vi "Single Tone Multi Ch Audio Measurements.vi"(8 "error in":errorcluster, 9 "units":T1, 10 "measurement settings":T3={"Band start"=20.0, "Band stop"=20000.0, "Amplitude"=1.0, "Frequency"=1000.0, "Full scale range"=3.16}, 11 "waveforms":waveform(dbl)[](array[waveform])) -> (0 "error out":errorcluster, 1 "spectra":cluster{"x0":dbl, "dx":dbl, "magnitude":dbl[]}[](array[cluster]), 2 "waveforms":waveform(dbl)[](array[waveform]), 3 "results":T2(array[cluster]))   [LabVIEW 2021]
uses:
  controls/Single Tone Measurement Settings.ctl
  controls/Single Tone Units.ctl
  <vilib>/addons/_NISVFA/_Shared subVIs/Common/SVL Set dB Reference (N Ch - 1 Ref).vi
  <vilib>/addons/Sound and Vibration/svt_Single Tone Measurements/SVT Spurious Free Dynamic Range (Frequency) (1 Ch).vi
  <vilib>/addons/_NISVFA/_Spectrum Processing/SVFA Unit Conversion (Complex) (1 Ch).vi
  <vilib>/addons/_NISVFA/_Spectrum Processing/SVFA Get Spectrum Subset (1 Ch).vi
  <vilib>/addons/_NISVFA/_Shared subVIs/Common/SVL Set dB Reference (1 Ch).vi
  <vilib>/addons/_NISVFA/_Spectrum Processing/SVFA Get Spectrum Subset (Complex) (1 Ch).vi
  <vilib>/addons/_NISVFA/_Shared subVIs/Common/svc_Window Parameters.vi
  <vilib>/addons/_NISVFA/_Shared subVIs/Common/svc_Extract Single Tone Information (complex).vi
  <vilib>/addons/_NISVFA/_Shared subVIs/Common/svc_Check Frequency Range in Spectrum.vi
  <vilib>/addons/_NISVFA/_Spectrum Processing/SVFA Spectrum Peak Search.vi
  <vilib>/addons/_NISVFA/_Spectrum Processing/SVFA Spectrum Peak Search (1 Ch).vi
  <vilib>/addons/_NISVFA/_Shared subVIs/Common/svc_Spectrum Units.vi
  <vilib>/addons/_NISVFA/_Shared subVIs/Common/svc_Log View for Spectrum (1Ch).vi
  <vilib>/addons/_NISVFA/_Spectrum Processing/SVFA Unit Conversion (1 Ch).vi
  <vilib>/addons/_NISVFA/_Shared subVIs/Common/svc_Complex Datatype Defaults.vi
  <vilib>/addons/_NISVFA/_Shared subVIs/Common/svc_Build Unit Label for Frequency Range.vi
  <vilib>/addons/_NISVFA/_Shared subVIs/Common/SVL Set dB Reference (variant).vi
  <vilib>/addons/_NISVFA/_Spectrum Processing/SVFA Get Tone Amplitude and Phase (1 Ch).vi
  <vilib>/addons/_NISVFA/_Spectrum Processing/subVIs/svfa_Compute Complex Spectrum for Export.vi
  <vilib>/addons/_NISVFA/_Shared subVIs/Common/svc_Check Frequency Range in Bandwidth.vi
  <vilib>/addons/_NISVFA/_Shared subVIs/Common/svc_Convert Start and Stop to Start Index and Length.vi
  <vilib>/addons/_NISVFA/_Spectrum Processing/subVIs/svfa_Spectrum Peak Search.vi
  <vilib>/addons/_NISVFA/_Shared subVIs/Common/svc_Format Value (DBL).vi
  <vilib>/addons/_NISVFA/_Shared subVIs/Common/svc_Get Weighting Enum and Labels.vi
  <vilib>/addons/_NISVFA/_Shared subVIs/Common/svc_Engineering Units to Unit Label.vi
  <vilib>/addons/_NISVFA/_Shared subVIs/Common/svc_Surround NonAlpha String with Parentheses.vi
  <vilib>/dlg_ctls.llb/Space Constant.vi
  <vilib>/addons/_NISVFA/_Shared subVIs/Common/svc_Unwrap Phase.vi
  <vilib>/addons/_NISVFA/_Shared subVIs/Common/svc_Convert Spectrum Array to dB.vi
  <vilib>/addons/_NISVFA/_Spectrum Processing/subVIs/svfa_Conversion Utility (spectrum info).vi
  <vilib>/addons/_NISVFA/_Spectrum Processing/subVIs/svfa_Window Frequency Response.vi
  <vilib>/addons/_NISVFA/_Spectrum Processing/subVIs/svfa_Window Frequency Response (double array).vi
  <vilib>/Analysis/baseanly.llb/Dot Product.vi
  <vilib>/Analysis/baseanly.llb/Complex Dot Product.vi
  <vilib>/addons/_NISVFA/_Spectrum Processing/subVIs/svfa_Peak Rough Search Indices.vi
  <vilib>/addons/_NISVFA/_Shared subVIs/Common/svc_Unit Label Lexical Class.vi
  <vilib>/addons/_NISVFA/_Spectrum Processing/subVIs/svfa_Peak to RMS to Peak2Peak.vi
  <vilib>/addons/_NISVFA/_Spectrum Processing/subVIs/svfa_Mag to Mag2.vi
  <vilib>/addons/_NISVFA/_Spectrum Processing/subVIs/svfa_Linear to dB.vi
  <vilib>/addons/_NISVFA/_Spectrum Processing/subVIs/svfa_dBrefA to dBrefB.vi
  <vilib>/addons/_NISVFA/_Spectrum Processing/subVIs/svfa_Spectrum to Spectral Density.vi
  <vilib>/addons/_NISVFA/_Spectrum Processing/subVIs/svfa_Rect Window Frequency Response.vi
  <vilib>/addons/_NISVFA/_Spectrum Processing/subVIs/svfa_Cosine Window Coefficients.vi
  <vilib>/addons/_NISVFA/_Shared subVIs/Common/svc_Caller VI Returned in Error Source.vi
  <vilib>/addons/Sound and Vibration/svt_Single Tone Measurements/SVT Gain (Time) (1 Ch).vi
  <vilib>/addons/Sound and Vibration/svt_Distortion/SVT SNR without Harmonics (Frequency) (1 Ch).vi
  <vilib>/addons/_NISVFA/_Spectrum Processing/SVFA Extract Single Tone Information (Complex) (1 Ch).vi
  <vilib>/addons/Sound and Vibration/svt_Single Tone Measurements/SVT Dynamic Range (Frequency) (1 Ch).vi
  <vilib>/addons/Sound and Vibration/svt_Distortion/subVIs/sv_Check Data Valid (Audio) (1 Ch).vi
  <vilib>/addons/_NISVFA/_Shared subVIs/Common/svc_Convert Frequency to Frequency String.vi
  <vilib>/Analysis/4window.llb/window parameters.vi
  <vilib>/Analysis/4window.llb/Window Properties.vi
  <vilib>/Analysis/4window.llb/Window Properties by Name.vi
  <vilib>/addons/_NISVFA/_Spectrum Processing/subVIs/svfa_Spectrum Peak Tone Search and Estimation (complex).vi
  <vilib>/measure/masignal.llb/Tones and Noise Waveform.vi
  <vilib>/addons/_NISVFA/_Shared subVIs/Common/svc_FFT with Window.vi
  <vilib>/Analysis/1siggen.llb/Square Wave.vi
  <vilib>/addons/_NISVFA/_Spectrum Processing/subVIs/svfa_Three Finger Peak Search.vi
  <vilib>/addons/Sound and Vibration/svt_Distortion/subVIs/sv_Peak View Amplitude (1 Ch).vi
  <vilib>/addons/Sound and Vibration/svt_Single Tone Measurements/SoundVib_SingleTone.lvlib
  <vilib>/addons/Sound and Vibration/svt_Distortion/SoundVib_Distortion.lvlib
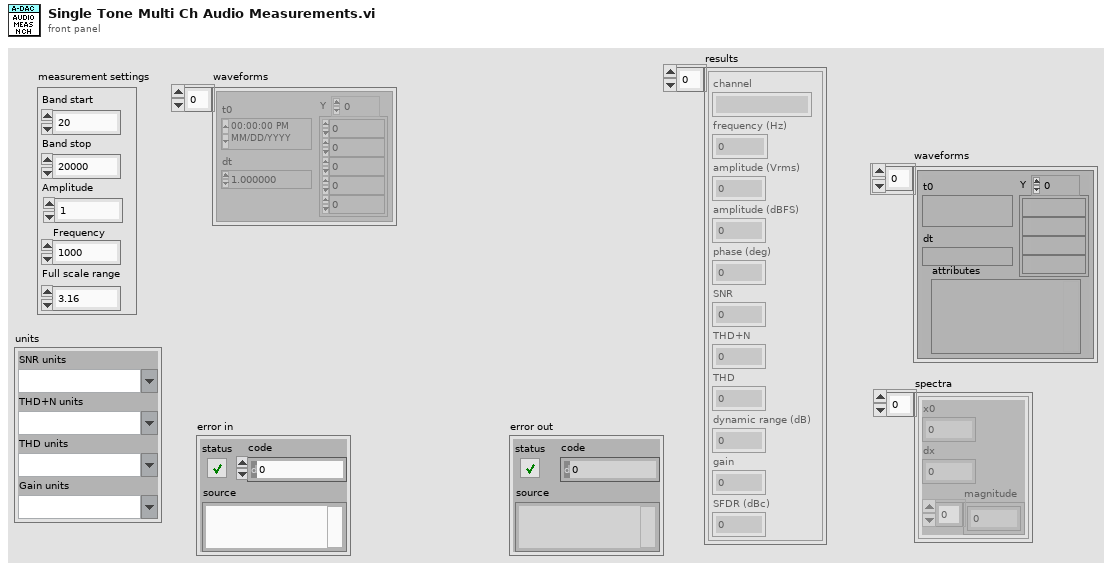
[diagram p1: front panel]
types:
  T1 = typedef "Single Tone Units.ctl" = cluster{"SNR units":string, "THD+N units":string, "THD units":string, "Gain units":string}
  T2 = cluster{"channel":string, "frequency (Hz)":dbl, "amplitude (Vrms)":dbl, "amplitude (dBFS)":dbl, "phase (deg)":dbl, "SNR":dbl, "THD+N":dbl, "THD":dbl, "dynamic range (dB)":dbl, "gain":dbl, "SFDR (dBc)":dbl}[]
  T3 = typedef "Single Tone Measurement Settings.ctl" = cluster{"Band start":dbl, "Band stop":dbl, "Amplitude":dbl, "Frequency":dbl, "Full scale range":dbl}
  T4 = cluster{"start frequency":dbl, "stop frequency":dbl}
  T5 = cluster{"SNR units":enum16{"dB", "linear ratio", "%"}, "detected fundamental amplitude units":enum16{"EU rms", "EU peak", "EU peak-peak"}}
  T6 = cluster{"gain units":enum16{"dB", "linear ratio"}, "detected fundamental amplitude units":enum16{"EU rms", "EU peak", "EU peak-peak"}}
  T7 = enum16{"no change", "spectrum", "spectral density"}
  T8 = cluster{"linear/dB":enum16{"no change", "linear", "dB"}, "dB reference (0: no change)":dbl, "power/magnitude":enum16{"no change", "power", "magnitude"}, "view":enum16{"no change", "rms", "peak", "peak-peak"}}
  T9 = cluster{"channel":string, "frequency (Hz)":dbl, "amplitude (Vrms)":dbl, "amplitude (dBFS)":dbl, "phase (deg)":dbl, "SNR":dbl, "THD+N":dbl, "THD":dbl, "dynamic range (dB)":dbl, "gain":dbl, "SFDR (dBc)":dbl}
  T10 = typedef "svc_Spectrum Info.ctl" = cluster{"channel name":string, "description":string, "x-axis units":T11, "spectral info":cluster{"spectrum type":T12, "linear/dB":enum16{"linear", "dB"}, "window":u16, "window size":i32, "FFT size":i32}, "engineering units":T13, "custom label":string, "dB reference [EU]":dbl, "peak units":enum16{"rms", "peak", "peak-peak"}, "weighting filter":T14, "spectral density?":bool, "unit label":string, "spectrum skewed?":bool, "complimentary spectrum units":T15}
  T11 = typedef "svc_X-Axis Units.ctl" = u16
  T12 = typedef "svc_Spectrum Type.ctl" = enum16{"FFT Spectrum [complex]", "Amplitude [Magnitude]", "Power [Magnitude^2]", "Cross Spectrum [complex]", "Frequency Response [Complex]"}
  T13 = typedef "svc_Engineering Units Text Ring.ctl" = u16
  T14 = typedef "svc_Weighting Filter Text Ring.ctl" = u16
  T15 = typedef "svc_Complimentary Spectrum Units.ctl" = enum16{"none", "radians", "degrees", "cycles", "imaginary"}
  T16 = cluster{"complex spectrum response":cluster{"f0":dbl, "df":dbl, "complex spectrum":cdb[]}, "spectrum info":T10}
  T17 = cluster{"frequency [Hz]":dbl, "amplitude [EU pk]":dbl, "phase (deg)":dbl}
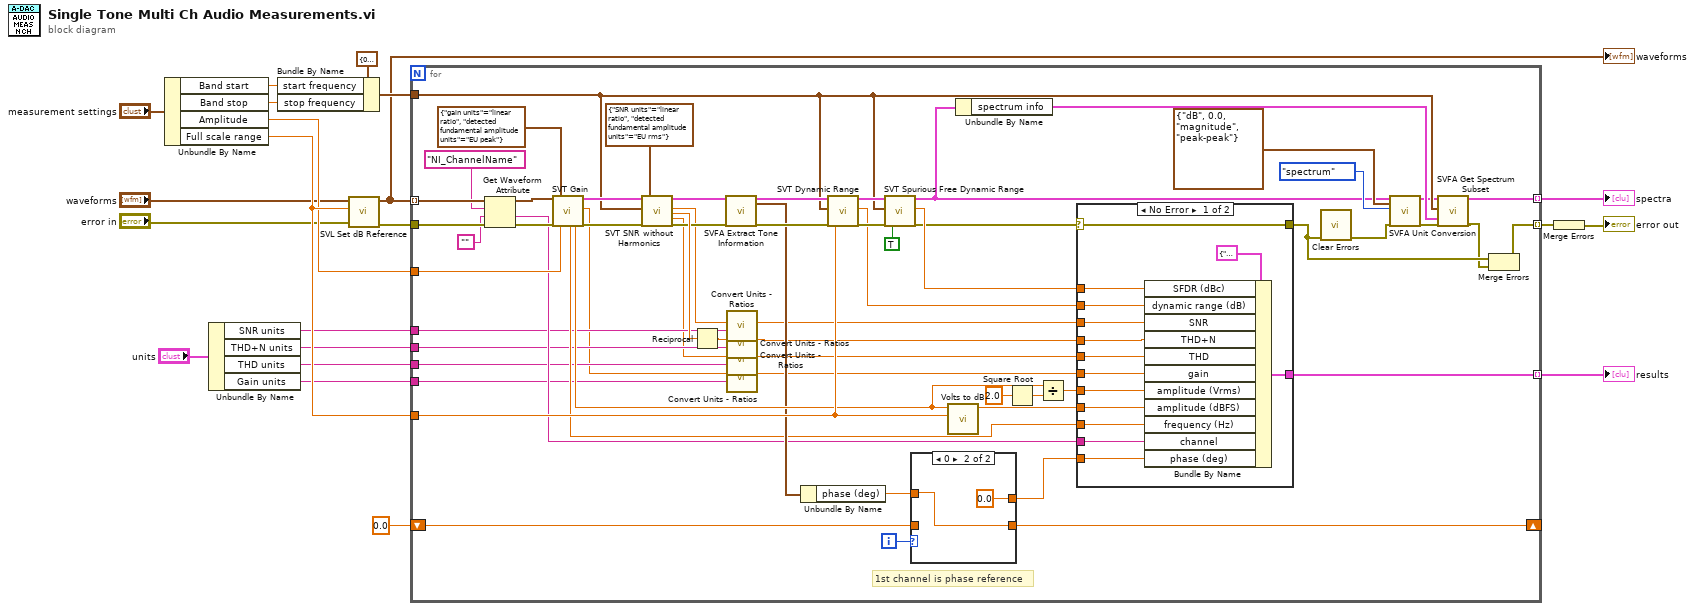
[diagram p0: block diagram]
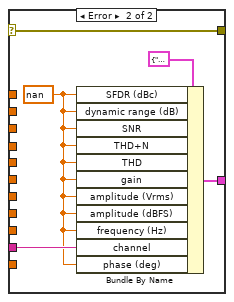
[diagram p2: hidden frame]
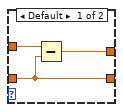
[diagram p3: hidden frame]
diagram:
  n1 = Unbundle By Name("measurement settings") -> ("Band start"=w20:dbl, "Band stop"=w21:dbl, "Amplitude"=w14:dbl, "Full scale range"=w16:dbl)
  n2 = Unbundle By Name("units") -> ("SNR units"=w4:string, "THD+N units"=w3:string, "THD units"=w2:string, "Gain units"=w1:string)
  n3 = Bundle By Name(cluster=T4 {"start frequency"=0.0, "stop frequency"=0.0} ("frequency range"), "start frequency"=w20, "stop frequency"=w21) -> (w18:T4)
  n4 = call-poly <vilib>:"SVL Set dB Reference.vi"("error in (no error)"="error in", "dB reference [EU]"=w16, "scaled signals in [EU]"="waveforms") -> ("error out"=w15:errorcluster, "scaled signals out [EU]"=w11:waveform(dbl)[])  [unwired: 7 in]
  "waveforms" <- w11
  n5 = for {
    tunnel: w18 -> [w26]
    tunnel: w16 -> [w73]
    tunnel: [w70] -> w9 mode=indexing
    tunnel: w14 -> [w69]
    tunnel: [w28] -> w8 mode=indexing
    tunnel: w11 -> [w53] mode=indexing
    shift-right: [w55] -> _
    shift-left: 0.0 -> [w57]
    tunnel: w15 -> [w51]
    tunnel: [w43] -> w6 mode=indexing
    tunnel: w4 -> [w40]
    tunnel: w3 -> [w37]
    tunnel: w2 -> [w34]
    tunnel: w1 -> [w31]
    i -> [w42]
    # "1st channel is phase reference"
    n6 = Get Waveform Attribute(4:w51, 5:"", 6:"NI_ChannelName" ("name"), 7:w53) -> (0:w50:errorcluster, 1:w47:string, 3:w52:waveform(dbl))  [unwired: 1 out]
    n7 = call-poly <vilib>:"SVT Gain.vi"("scaled signal [EU]"=w52, "error in (no error)"=w50, "desired units"=T6 {"gain units"=enum."linear ratio", "detected fundamental amplitude units"=enum."EU peak"}, "amplitude [EU peak]"=w69) -> ("detected fundamental\nfrequency [Hz]"=w41:dbl, "detected fundamental\namplitude"=w63:dbl, "complex spectrum"=w76:T16, "gain"=w30:dbl, "error out"=w77:errorcluster)  [unwired: 10 in, 1 out]
    n8 = call-poly <vilib>:"SVT SNR without Harmonics.vi"("complex spectrum"=w76, "frequency range"=w26, "error in (no error)"=w77, "desired units"=T5 {"SNR units"=enum."linear ratio", "detected fundamental amplitude units"=enum."EU rms"}) -> ("complex spectrum"=w62:T16, "SNR (without harmonics)"=w39:dbl, "SINAD"=w68:dbl, "THD"=w33:dbl, "error out"=w61:errorcluster)  [unwired: 8 in, 3 out]
    n9 = Reciprocal(x=w68) -> (1/x=w36:dbl)
    n10 = call-poly <vilib>:"SVFA Extract Tone Information.vi"("complex spectrum"=w62, "error in"=w61) -> ("complex spectrum"=w60:T16, "detected tone"=w58:T17, "error out"=w59:errorcluster)  [unwired: 14 in, 1 out]
    n11 = call "Convert Units - Ratios.vi"("units"=w40, "linear ratio"=w39) -> ("converted ratio"=w38:dbl)  [unwired: 9 in]
    n12 = call "Convert Units - Ratios.vi"("units"=w37, "linear ratio"=w36) -> ("converted ratio"=w35:dbl)  [unwired: 9 in]
    n13 = call "Convert Units - Ratios.vi"("units"=w34, "linear ratio"=w33) -> ("converted ratio"=w32:dbl)  [unwired: 9 in]
    n14 = call "Convert Units - Ratios.vi"("units"=w31, "linear ratio"=w30) -> ("converted ratio"=w29:dbl)  [unwired: 9 in]
    n15 = Unbundle By Name(w58) -> ("phase (deg)"=w56:dbl)
    n16 = call-poly <vilib>:"SVT Dynamic Range.vi"("complex spectrum"=w60, "frequency range"=w26, "error in (no error)"=w59, "full scale amplitude [EU peak]"=w73) -> ("dup complex spectrum"=w80:T16, "dynamic range"=w71:dbl, "error out"=w81:errorcluster)  [unwired: 10 in, 3 out]
    n17 = call-poly <vilib>:"SVT Spurious Free Dynamic Range.vi"("complex spectrum"=w80, "frequency range"=w26, "error in (no error)"=w81, "exclude harmonics"=TRUE) -> ("complex spectrum"=w25:T16, "spurious free dynamic range"=w72:dbl, "error out"=w46:errorcluster)  [unwired: 8 in, 5 out]
    n18 = case shown="0" w42 {
      tunnel: w57 -> [w103 _]
      tunnel: w56 -> [w104 w106]
      tunnel: [w102 0.0] -> w54
      tunnel: [w103 w106] -> w55
      frame Default {
        n19 = Subtract(x=w104, y=w103) -> (x-y=w102:dbl)
      }
      frame 0 {
      }
    }
    n20 = call "Volts to dB.vi"("Full scale range"=w73, "Voltage(V)"=w63) -> ("Voltage(dB)"=w67:dbl)  [unwired: 9 in]
    n21 = Unbundle By Name(w25) -> ("spectrum info"=w24:T10)
    n22 = Square Root(x=2.0 ("y")) -> (sqrt(x)=w66:dbl)
    n23 = Divide(x=w63, y=w66) -> (x/y=w64:dbl)
    n24 = case shown="No Error" w46 {
      selector: w46 -> [w83 w97]
      tunnel: w72 -> [w96 _]
      tunnel: w71 -> [w95 _]
      tunnel: [w93 w100] -> w70
      tunnel: w29 -> [w92 _]
      tunnel: w38 -> [w91 _]
      tunnel: w35 -> [w90 _]
      tunnel: w32 -> [w89 _]
      tunnel: w41 -> [w88 _]
      tunnel: w67 -> [w87 _]
      tunnel: w64 -> [w86 _]
      tunnel: w54 -> [w85 _]
      tunnel: w47 -> [w84 w99]
      tunnel: [w83 w97] -> w44
      frame No Error {
        n25 = Bundle By Name(cluster=T9 {"channel"="", "frequency (Hz)"=0.0, "amplitude (Vrms)"=0.0, "amplitude (dBFS)"=0.0, "phase (deg)"=0.0, "SNR"=0.0, "THD+N"=0.0, "THD"=0.0, "dynamic range (dB)"=0.0, "gain"=0.0, "SFDR (dBc)"=0.0} ("results"), "SFDR (dBc)"=w96, "dynamic range (dB)"=w95, "SNR"=w91, "THD+N"=w90, "THD"=w89, "gain"=w92, "amplitude (Vrms)"=w86, "amplitude (dBFS)"=w87, "frequency (Hz)"=w88, "channel"=w84, "phase (deg)"=w85) -> (w93:T9)
      }
      frame Error {
        w98 = nan ("SFDR (dBc)")
        n26 = Bundle By Name(cluster=T9 {"channel"="", "frequency (Hz)"=0.0, "amplitude (Vrms)"=0.0, "amplitude (dBFS)"=0.0, "phase (deg)"=0.0, "SNR"=0.0, "THD+N"=0.0, "THD"=0.0, "dynamic range (dB)"=0.0, "gain"=0.0, "SFDR (dBc)"=0.0} ("results"), "SFDR (dBc)"=w98, "dynamic range (dB)"=w98, "SNR"=w98, "THD+N"=w98, "THD"=w98, "gain"=w98, "amplitude (Vrms)"=w98, "amplitude (dBFS)"=w98, "frequency (Hz)"=w98, "channel"=w99, "phase (deg)"=w98) -> (w100:T9)
      }
    }
    n27 = call <vilib>:"Clear Errors.vi"("error in (no error)"=w44) -> ("error out"=w45:errorcluster)  [unwired: 5 in, 1 out]
    n28 = call-poly <vilib>:"SVFA Unit Conversion.vi"("complex spectrum"=w25, "desired scaling"=T8 {"linear/dB"=enum."dB", "dB reference (0: no change)"=0.0, "power/magnitude"=enum."magnitude", "view"=enum."peak-peak"}, "spectral density desired"=T7."spectrum", "error in (no error)"=w45) -> ("converted spectrum"=w22:cluster{"x0":dbl, "dx":dbl, "magnitude":dbl[]}, "error out"=w23:errorcluster)  [unwired: 10 in, 4 out]
    n29 = call-poly <vilib>:"SVFA Get Spectrum Subset.vi"("spectrum"=w22, "range"=w26, "spectrum info"=w24, "error in (no error)"=w23) -> ("spectrum subset"=w28:cluster{"x0":dbl, "dx":dbl, "magnitude":dbl[]}, "error out"=w27:errorcluster)  [unwired: 10 in, 4 out]
    n30 = Merge Errors(w44, w27) -> (w43:errorcluster)
  }
  "results" <- w9
  "spectra" <- w8
  n31 = Merge Errors(w6) -> (→"error out":errorcluster)
